vi "BlackBox_filtered _1d.vi"() -> ()   [LabVIEW 2019]
uses:
  <vilib>/Analysis/Matrix/Datatypes/RealMatrix.ctl
  <vilib>/userDefined/High Color/IMAQdx.ctl
  <vilib>/Platform/TimedLoop/XDataNode/timing_clust.ctl
  <vilib>/Platform/TimedLoop/XDataNode/nitl_modes.ctl
  <vilib>/Platform/TimedLoop/XDataNode/wakeup.ctl
  <vilib>/myRIO/Instrument Drivers/Onboard IO/AO/typedefs/AO Reference.ctl
  <vilib>/myRIO/Common/Instrument Driver Framework/Utilities/typedefs/myRIO Generic Hardware Reference.ctl
  <vilib>/myRIO/Common/Instrument Driver Framework/Utilities/typedefs/Hardware Version Enum.ctl
  <vilib>/myRIO/Common/Instrument Driver Framework/Utilities/typedefs/myRIO v1.0 Reference.ctl
  <vilib>/myRIO/Common/Instrument Driver Framework/Utilities/typedefs/Generic FPGA Reference.ctl
  <vilib>/myRIO/Common/Instrument Driver Framework/myRIO v1.0/AO/typedefs/AO Channels List.ctl
  <vilib>/myRIO/Common/Instrument Driver Framework/myRIO v1.0/AO/typedefs/AO Channels Enum.ctl
  <vilib>/myRIO/Common/Instrument Driver Framework/Utilities/typedefs/Analog Scaling Constants List.ctl
  <vilib>/myRIO/Common/Instrument Driver Framework/Utilities/typedefs/Analog Scaling Constants.ctl
  <vilib>/userDefined/High Color/nirio_resource_hc.ctl
  <vilib>/myRIO/Common/Instrument Driver Framework/myRIO v1.0/Encoder/typedefs/Encoder Signal Mode.ctl
  <vilib>/myRIO/Instrument Drivers/Onboard IO/Encoder/typedefs/Encoder Reference.ctl
  <vilib>/myRIO/Common/Instrument Driver Framework/myRIO v1.0/Encoder/typedefs/Encoder Channels Enum.ctl
  <vilib>/myRIO/Common/Instrument Driver Framework/myRIO v1.0/Encoder/typedefs/Encoder Configuration v1.0.ctl
  <vilib>/myRIO/Common/Instrument Driver Framework/Utilities/vis/Is FPGA Ref Available.vi
  <vilib>/myRIO/Common/Instrument Driver Framework/myRIO v1.0/AO/vis/myRIO v1.1 Open AO.vi
  <vilib>/myRIO/Instrument Drivers/Onboard IO/AO/vis/Write.vi
  <vilib>/myRIO/Common/Instrument Driver Framework/myRIO v1.0/Encoder/vis/myRIO v1.1 Open Encoder.vi
  <vilib>/myRIO/Instrument Drivers/Onboard IO/Encoder/vis/Read.vi
  <vilib>/myRIO/Common/Instrument Driver Framework/Utilities/vis/Validate Channels.vi
  <vilib>/myRIO/Common/Instrument Driver Framework/myRIO v1.0/AO/vis/myRIO v1.0 Reserve AO.vi
  <vilib>/myRIO/Common/Instrument Driver Framework/myRIO v1.0/Encoder/vis/myRIO v1.0 Reserve Encoder.vi
  <vilib>/Analysis/baseanly.llb/A x B.vi
  <vilib>/Analysis/baseanly.llb/A x Vector.vi
  <vilib>/myRIO/Common/Instrument Driver Framework/myRIO v1.0/AO/vis/myRIO v1.0 Build MUX Configuration AO.vi
  <vilib>/myRIO/Common/Instrument Driver Framework/myRIO v1.0/Resource Manager/vis/myRIO v1.0 Reserve Channel List.vi
  <vilib>/myRIO/Common/Instrument Driver Framework/myRIO v1.0/Encoder/vis/myRIO v1.0 Build MUX Configuration Encoder.vi
  <vilib>/myRIO/Common/Instrument Driver Framework/myRIO v1.0/Resource Manager/vis/myRIO v1.0 Reserve Channel.vi
  <vilib>/myRIO/Common/Instrument Driver Framework/myRIO v1.0/Resource Manager/vis/myRIO v1.0 Unreserve Channel.vi
  <vilib>/myRIO/Common/Instrument Driver Framework/myRIO v1.0/Resource Manager/vis/myRIO v1.0 Create Configuration List.vi
  <vilib>/myRIO/Common/Instrument Driver Framework/myRIO v1.0/Resource Manager/vis/myRIO v1.0 Build Mutex Name.vi
  <vilib>/Utility/VariantDataType/GetNumericInfo.vi
  <vilib>/Utility/error.llb/Error Cluster From Error Code.vi
  <vilib>/myRIO/Common/Instrument Driver Framework/myRIO v1.0/myRIO v1.1 Open.vi
  <vilib>/myRIO/Common/Instrument Driver Framework/myRIO v1.0/AO/vis/myRIO v1.0 Get Scaling Constants AO.vi
  <vilib>/myRIO/Common/Instrument Driver Framework/Utilities/vis/IO Manager.vi
  <vilib>/myRIO/Common/Instrument Driver Framework/Utilities/vis/Configuration Manager.vi
  <vilib>/myRIO/Common/Instrument Driver Framework/myRIO v1.0/myRIO v1.0 Close.vi
  <vilib>/myRIO/Common/Instrument Driver Framework/myRIO v1.0/AO/vis/myRIO v1.0 Write AO.vi
  <vilib>/Utility/file.llb/Write Delimited Spreadsheet (DBL).vi
  <vilib>/myRIO/Common/Instrument Driver Framework/myRIO v1.0/Resource Manager/vis/myRIO v1.0 Configure IO.vi
  <vilib>/myRIO/Common/Instrument Driver Framework/myRIO v1.0/Encoder/vis/myRIO v1.0 Configure Encoder.vi
  <vilib>/myRIO/Common/Instrument Driver Framework/myRIO v1.0/Encoder/vis/myRIO v1.0 Read Encoder.vi
  <vilib>/platform/TimedLoop/XDataNode/XDataNode.xnode
  <vilib>/myRIO/Express VI/Onboard IO/AO/AO Express VI.xnode
  <vilib>/myRIO/Instrument Drivers/Onboard IO/AO/vis/myRIO AO Open.xnode
  <vilib>/myRIO/Express VI/Onboard IO/Encoder/Encoder Express VI.xnode
  <vilib>/myRIO/Instrument Drivers/Onboard IO/Encoder/vis/myRIO Encoder Open.xnode
  <vilib>/myRIO/Common/Instrument Driver Framework/myRIO v1.0/Encoder/typedefs/Encoder Count Direction Enum.ctl
  <vilib>/Platform/TimedLoop/XDataNode/XDNodeRunTimeDep.lvlib
  <vilib>/myRIO/Instrument Drivers/Onboard IO/AO/AO.lvlib
  <vilib>/vision/driver/NI_Vision_Acquisition_Software.lvlib
  <vilib>/myRIO/Instrument Drivers/Onboard IO/Encoder/Encoder.lvlib
  <vilib>/vision/NI_Vision_Development_Module.lvlib
  <vilib>/Analysis/Matrix/NI_Matrix.lvlib
panel:
  out "scaled_obs_y":dbl[](array[numeric])
  out "scaled_obs_x":dbl[](array[numeric])
  out "done":bool
  out "target_y":dbl
  out "target_x":dbl
  in  "start_test":bool
  out "observation":dbl[](array[numeric])
  out "scaled_obs":dbl[](array[numeric])
  in  "record_name":string
  out "record":T1
  out "step_recorded":dbl
  in  "stop_recording":bool
  in  "start_recording":bool
  out "recording":bool
  out "record_t":dbl[](array[numeric])
  out "target_a_y":dbl(knob) scale=-45.0..45.0
  out "target_a_x":dbl(knob) scale=-45.0..45.0
  out "y_angle":dbl(knob) scale=-45.0..45.0
  out "x_angle":dbl(knob) scale=-45.0..45.0
  out "y_error":dbl
  out "x_error":dbl
  out "y":dbl
  out "x":dbl
  out "camera":T2(plugin-control)
  in  "threshold":cluster{"Lower value":sgl, "Upper value":sgl}={"Lower value"=60.0, "Upper value"=255.0} {"Upper value" format="%.2f"; "Lower value" format="%.2f"}
  out "threshold":T2(plugin-control)
  out "x-y":u32
  out "y_input":dbl
  out "y_angle_error":dbl
  out "x_angle_error":dbl
  in  "stop":bool
  out "x_input":dbl
  in  "reset":bool
  in  "dt":dbl=20.0
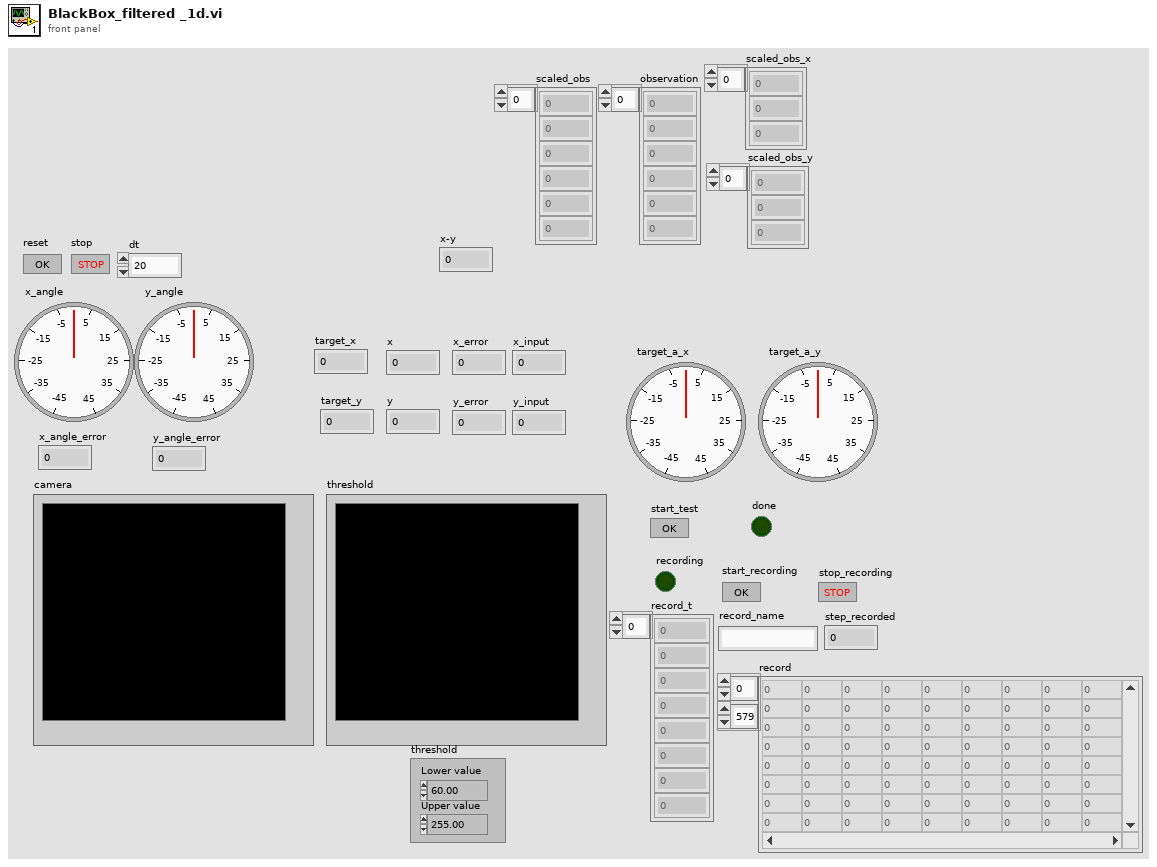
[diagram p1: front panel]
types:
  T1 = typedef "NI_Matrix.lvlib/RealMatrix.ctl" = dbl[][]
  T2 = typedef "IMAQ Image.ctl" = refnum<image>
  T3 = typedef "IMAQdx.ctl" = refnum<k21>
  T4 = typedef "XDNodeRunTimeDep.lvlib/timing_clust.ctl" = cluster{"Expected End [f-1]":u64, "Actual End [f-1]":u64, "Finished Late? [f-1]":bool, "Expected End [i-1]":u64, "Actual End [i-1]":u64, "Finished Late? [i-1]":bool, "Expected Start [i]":u64, "Actual Start [i]":u64, "Expected Start [f]":u64, "Actual Start [f]":u64, "Source Name":string, "Structure Name":string, "Period":i64, "Deadline":i64, "Offset":i64, "Start":i64, "Priority":i32, "Timeout":i32, "Mode":T5, "Wakeup Reason":T6, "Error":errorcluster, "Source Type":string, "Secondary Source Type":string, "Global End Time":u64, "Global Start Time":u64, "Frame Duration":u64, "Iteration Duration":u64, "Assigned CPU":i32, "I/O Scan Engine Mode":u32}
  T5 = typedef "XDNodeRunTimeDep.lvlib/nitl_modes.ctl" = enum32{"No Change", "Process missed periods, maintain original phase", "Discard missed periods, maintain original phase", "Process missed periods, ignore original phase", "Discard missed periods, ignore original phase"}
  T6 = typedef "XDNodeRunTimeDep.lvlib/wakeup.ctl" = enum32{"Normal", "Aborted", "Asynchronous wakeup", "Timing source error", "Timed loop error", "Timeout"}
  T7 = typedef "Encoder.lvlib/Encoder Reference.ctl" = cluster{"myRIO Reference":T8, "Encoder Channels Enum":T12}
  T8 = typedef "myRIO Generic Hardware Reference.ctl" = cluster{"myRIO Model":T9, "myRIO Hardware Reference":T10}
  T9 = typedef "Hardware Version Enum.ctl" = enum16{"Unknown", "myRIO-1900", "myRIO-1950", "roboRIO", "NI ELVIS RIO CM", "ELVIS III"}
  T10 = typedef "myRIO v1.0 Reference.ctl" = cluster{"Generic FPGA Reference":T11, "Allow multiple opens":bool}
  T11 = typedef "Generic FPGA Reference.ctl" = refnum<k20>
  T12 = typedef "Encoder Channels Enum.ctl" = enum16{"Not Connected", "C/ENC0", "C/ENC1", "A/ENC", "A/ENC0", "A/ENC1", "A/ENC2", "A/ENC3", "A/ENC4", "A/ENC5", "A/ENC6", "A/ENC7", "A/ENC8", "A/ENC9", "B/ENC", "B/ENC0", "B/ENC1", "B/ENC2", "B/ENC3", "B/ENC4", "B/ENC5", "B/ENC6", "B/ENC7", "B/ENC8", "B/ENC9", "DIO/ENC0", "DIO/ENC1", "DIO/ENC2", "DIO/ENC3", "DIO/ENC4"}
  T13 = typedef "Encoder Signal Mode.ctl" = enum16{"Quadrature phase signal", "Step and direction signal"}
  T14 = typedef "nirio_resource_hc.ctl" = tag
  T15 = typedef "AO.lvlib/AO Reference.ctl" = cluster{"myRIO Reference":T8, "AO Channel List":T16, "AO Scaling Constant List":T18}
  T16 = typedef "AO Channels List.ctl" = T17[]
  T17 = typedef "AO Channels Enum.ctl" = enum16{"Not Connected", "AudioOut/Left", "AudioOut/Right", "C/AO0", "C/AO1", "A/AO0", "A/AO1", "B/AO0", "B/AO1"}
  T18 = typedef "Analog Scaling Constants List.ctl" = T19[]
  T19 = typedef "Analog Scaling Constants.ctl" = cluster{"LSB Weight (Volts)":dbl, "Offset (Volts)":dbl, "Signed?":bool}
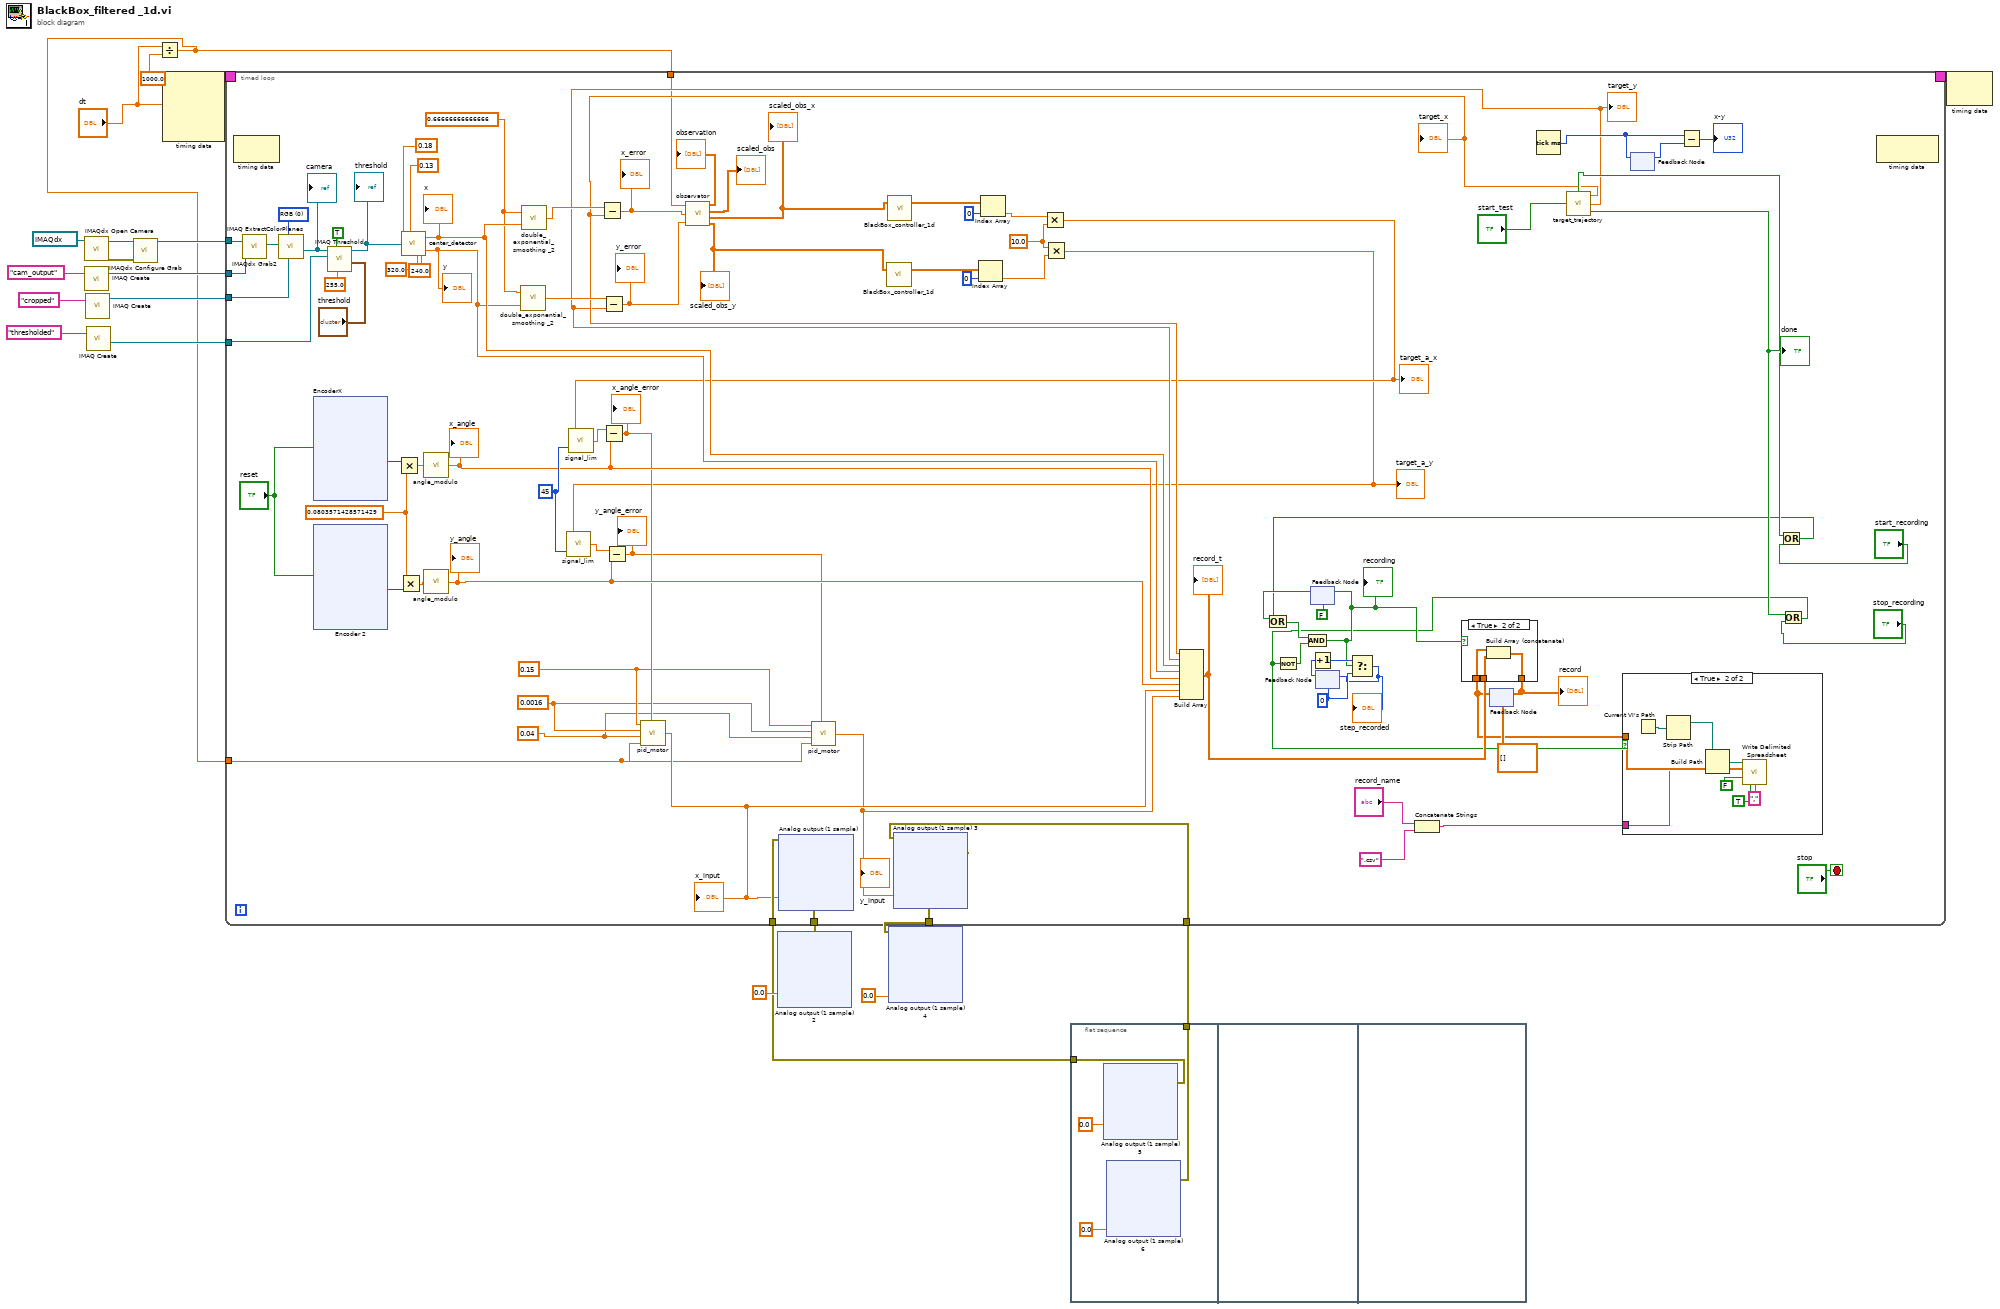
[diagram p0: block diagram]
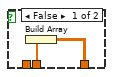
[diagram p3: hidden frame]
diagram:
  n1 = call <vilib>:"IMAQdx Open Camera.vi"("Session In"=T3 "cam2") -> ("error out"=w13:errorcluster, "Session Out"=w14:T3)  [unwired: 9 in]
  n2 = call "IMAQ Create"("Image Name"="cam_output") -> ("New Image"=w15:T2)  [unwired: 4 in, 1 out]
  n3 = call "IMAQ Create"("Image Name"="cropped") -> ("New Image"=w6:T2)  [unwired: 4 in, 1 out]
  n4 = call "IMAQ Create"("Image Name"="thresholded") -> ("New Image"=w4:T2)  [unwired: 4 in, 1 out]
  n5 = call <vilib>:"IMAQdx Configure Grab.vi"("error in"=w13, "Session In"=w14) -> ("Session Out"=w16:T3)  [unwired: 8 in, 1 out]
  n6 = Divide(x="dt", y=1000.0) -> (x/y=w1:dbl)
  n7 = node-c288("dt") -> (w21:T4)  [unwired: 3 in]
  n8 = timed-loop {
    timing: w21 -> [_]
    timing-out: [_] -> w20
    tunnel: w16 -> [w109]
    tunnel: w15 -> [w108]
    tunnel: w1 -> [w50]
    tunnel: [w97] -> w11
    tunnel: [w93] -> w10
    tunnel: w9 -> [w92]
    tunnel: w8 -> [w91]
    tunnel: w6 -> [w66]
    tunnel: w4 -> [w60]
    tunnel: w1 -> [w38]
    stop <- "stop" stop-if-true
    w24 = 10.0
    w55 = 0.66666666666666
    w47 = 0.04 ("ki")
    w48 = 0.0016 ("kd")
    w49 = 0.15 ("kp")
    w69 = u16 0 items=["RGB", "HSL", "HSV", "HSI"] ("Color Mode")
    w79 = 0
    w98 = 45
    w106 = 0.0803571428571429
    n9 = node-c288() -> ()  [unwired: 1 in, 1 out]
    n10 = call <vilib>:"IMAQdx Grab2.vi"("Image In"=w108, "Session In"=w109) -> ("Image Out"=w68:T2)  [unwired: 6 in, 3 out]
    n11 = call "IMAQ ExtractColorPlanes"("Blue or Luma or Val or Inten Plane"=w66, "Color Mode"=w69, "Image Src"=w68) -> ("Blue or Luma or Val or Inten Plane out"=w67:T2)  [unwired: 5 in, 3 out]
    "camera" <- w67
    n12 = xnode "EncoderX"("Reset Counter"="reset") -> ("Counter Value"=w107:i32)  [unwired: 1 in, 3 out]
    n13 = xnode "Encoder 2"("Reset Counter"="reset") -> ("Counter Value"=w105:i32)  [unwired: 1 in, 3 out]
    n14 = call "IMAQ Threshold"("Replace Value"=sgl 255.0, "Keep/Replace Value (Replace)"=TRUE, "Range"="threshold", "Image Dst"=w60, "Image Src"=w67) -> ("Image Dst Out"=w63:T2)  [unwired: 5 in, 1 out]
    "threshold" <- w63
    n15 = Multiply(x=w107, y=w106) -> (x*y=w102:dbl)
    n16 = Multiply(x=w106, y=w105) -> (x*y=w101:dbl)
    n17 = call "center_detector.vi"("px_x"=320.0, "px_y"=240.0, "Image"=w63, "m_x"=0.18, "m_y"=0.13) -> ("x"=w58:dbl, "y"=w56:dbl)
    "x" <- w58
    "y" <- w56
    n18 = call "angle_modulo.vi"("alpha"=w102) -> ("alpha_prime"=w87:dbl)
    "x_angle" <- w87
    n19 = call "angle_modulo.vi"("alpha"=w101) -> ("alpha_prime"=w86:dbl)
    "y_angle" <- w86
    n20 = call "double_exponential_smoothing _2.vi"("x"=w56, "alpha"=w55) -> ("dema"=w57:dbl)
    n21 = call "double_exponential_smoothing _2.vi"("x"=w58, "alpha"=w55) -> ("dema"=w59:dbl)
    n22 = feedback #1(FALSE) -> (w85:bool)
    n23 = feedback #2(w79) -> (w81:i32)
    n24 = Increment(x=w81) -> (x+1=w80:i32)
    n25 = Concatenate Strings("record_name", ".csv") -> (w70:string)
    n26 = feedback #3(T1 [] ("Real Matrix")) -> (w73:T1)
    n27 = Tick Count (ms)() -> (millisecond timer value=w96:u32)
    n28 = call "target_trajectory.vi"("start_test"="start_test") -> ("start"=w43:bool, "target_x"=w40:dbl, "target_y"=w39:dbl, "done"=w44:bool)
    "target_x" <- w40
    "target_y" <- w39
    "done" <- w44
    n29 = Subtract(x=w59, y=w40) -> (x-y=w37:dbl)
    "x_error" <- w37
    n30 = Subtract(x=w57, y=w39) -> (x-y=w36:dbl)
    "y_error" <- w36
    n31 = call "observator.vi"("d_t"=w38, "e_x"=w37, "e_y"=w36) -> ("observation"=→"observation":dbl[], "scaled_obs"=→"scaled_obs":dbl[], "scaled_obs_x"=w32:dbl[], "scaled_obs_y"=w31:dbl[])
    "scaled_obs_x" <- w32
    "scaled_obs_y" <- w31
    n32 = call "BlackBox_controller_1d.vi"("Normalized observation"=w31) -> ("output"=w27:dbl[])  [unwired: 1 in, 1 out]
    n33 = call "BlackBox_controller_1d.vi"("Normalized observation"=w32) -> ("output"=w30:dbl[])  [unwired: 1 in, 1 out]
    n34 = Index Array(array=w27, index=0) -> (element=w25:dbl)
    n35 = Index Array(array=w30, index=0) -> (element=w28:dbl)
    n36 = Multiply(x=w28, y=w24) -> (x*y=w23:dbl)
    "target_a_x" <- w23
    n37 = call "signal_lim.vi"("lim"=w98, "x"=w23) -> ("y"=w100:dbl)
    n38 = Subtract(x=w100, y=w87) -> (x-y=w54:dbl)
    "x_angle_error" <- w54
    n39 = call "pid_motor.vi"("kp"=w49, "kd"=w48, "ki"=w47, "dt"=w50, "err"=w54) -> ("u"=w53:dbl)
    "x_input" <- w53
    n40 = xnode "Analog output (1 sample)"("C/AO0 (AO0)"=w53, "error in (no error)"=w92) -> ("error out"=w97:errorcluster)
    n41 = Multiply(x=w24, y=w25) -> (x*y=w22:dbl)
    "target_a_y" <- w22
    n42 = call "signal_lim.vi"("lim"=w98, "x"=w22) -> ("y"=w99:dbl)
    n43 = Subtract(x=w99, y=w86) -> (x-y=w52:dbl)
    "y_angle_error" <- w52
    n44 = call "pid_motor.vi"("kp"=w49, "kd"=w48, "ki"=w47, "dt"=w50, "err"=w52) -> ("u"=w51:dbl)
    "y_input" <- w51
    n45 = xnode "Analog output (1 sample) 3"("C/AO1 (AO1)"=w51, "error in (no error)"=w91) -> ("error out"=w93:errorcluster)
    n46 = Build Array(w40, w39, w58, w56, w87, w86, w53, w51) -> (w76:dbl[])
    "record_t" <- w76
    n47 = feedback-in #4(w96) -> ()
    n48 = feedback #4() -> (w95:u32)  [unwired: 1 in]
    n49 = Subtract(x=w96, y=w95) -> (x-y=→"x-y":u32)
    n50 = Or(x=w43, y="start_recording") -> (x .or. y?=w42:bool)
    n51 = Or(x=w85, y=w42) -> (x .or. y?=w84:bool)
    n52 = Or(x=w44, y="stop_recording") -> (x .or. y?=w33:bool)
    n53 = Not(x=w33) -> (.not. x?=w83:bool)
    n54 = And(x=w84, y=w83) -> (x .and. y?=w77:bool)
    "recording" <- w77
    n55 = feedback-in #1(w77) -> ()
    n56 = Select(t=w80, s=w77, f=w79) -> (s? t:f=w78:i32)
    "step_recorded" <- w78
    n57 = feedback-in #2(w78) -> ()
    n58 = case shown="True" w77 {
      tunnel: w73 -> [_ w122]
      tunnel: [w118 w121] -> w74
      tunnel: w76 -> [w119 w120]
      frame False {
        n59 = Build Array(w119) -> (w118:T1)
      }
      frame True {
        n60 = Build Array (concatenate)(w122, w120) -> (w121:T1)
      }
    }
    "record" <- w74
    n61 = feedback-in #3(w74) -> ()
    n62 = case shown="True" w33 {
      tunnel: w73 -> [_ w117]
      tunnel: w70 -> [_ w115]
      frame False {
      }
      frame True {
        n63 = Current VI's Path() -> (path=w113:path)
        n64 = Strip Path(path=w113) -> (stripped path=w112:path)  [unwired: 1 out]
        n65 = Build Path(base path=w112, name or relative path=w115) -> (appended path=w114:path)
        n66 = call-poly <vilib>:"Write Delimited Spreadsheet.vi"("file path (dialog if empty)"=w114, "2D data"=w117, "append to file? (new file:F)"=FALSE, "transpose? (no:F)"=TRUE, "delimiter (\\t)"="," ("delimiter (\\t)")) -> ()  [unwired: 9 in, 2 out]
      }
    }
    n67 = node-c288() -> ()  [unwired: 1 in, 1 out]
  }
  n68 = xnode "Analog output (1 sample) 2"("C/AO0 (AO0)"=0.0, "error in (no error)"=w11) -> ()  [unwired: 1 out]
  n69 = xnode "Analog output (1 sample) 4"("C/AO1 (AO1)"=0.0, "error in (no error)"=w10) -> ()  [unwired: 1 out]
  n70 = flat-sequence {
    tunnel: [w292] -> w9
    tunnel: [w291] -> w8
    frame #0 {
      n71 = xnode "Analog output (1 sample) 5"("C/AO0 (AO0)"=0.0) -> ("error out"=w292:errorcluster)  [unwired: 1 in]
      n72 = xnode "Analog output (1 sample) 6"("C/AO1 (AO1)"=0.0) -> ("error out"=w291:errorcluster)  [unwired: 1 in]
    }
    frame #1 {
    }
    frame #2 {
    }
  }
  n73 = node-c288(w20) -> ()  [unwired: 1 out]
